vi "GigE Vision Set Packet Size.vi"(8 "error in (no error)":errorcluster, 10 "Packet Size":i32, 11 "Camera in":refnum<class "Camera.lvclass">) -> (0 "error out":errorcluster, 3 "Camera":refnum<class "Camera.lvclass">)   [LabVIEW 2020, in "Camera.lvclass"]
doc: "Specifies the stream packet size, in bytes, to send on the selected channel for a GVSP transmitter or specifies the maximum packet size supported by a GVSP receiver.\n\nThis does not include data leader and data trailer and the last data packet which might be of smaller size (since packet size is not necessarily a multiple of block size for stream channel). Negative packet_size is ignored."
uses:
  Camera.lvclass
  Camera.lvclass/Camera.ctl
  bin/gindustrialcam_32-1.dll
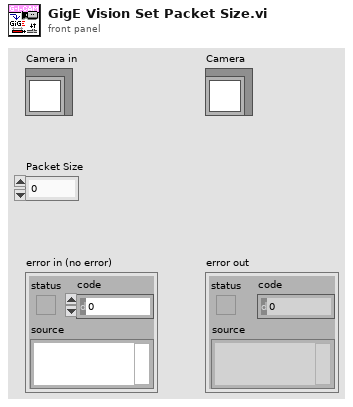
[diagram p1: front panel]
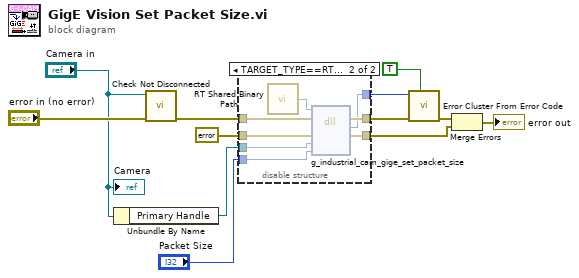
[diagram p0: block diagram]
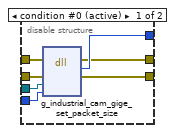
[diagram p2: hidden frame]
diagram:
  n1 = Unbundle By Name("Camera in") -> ("Primary Handle"=w2:refnum<data-value>)
  n2 = call "Check Not Disconnected.vi"("error in (no error)"="error in (no error)", "Camera in"="Camera in") -> ("error out"=w10:errorcluster)  [unwired: 9 in]
  n3 = disable-structure shown="TARGET_TYPE==RT&&OS==Linux" {
    disable-tunnel: w10 -> [w19 w26]
    disable-tunnel: errorcluster {"status"=FALSE, "code"=0, "source"=""} ("error constant") -> [w18 w25]
    disable-tunnel: [w17 w20] -> w7
    disable-tunnel: [w16 w21] -> w5
    disable-tunnel: [w15 w22] -> w4
    disable-tunnel: w2 -> [w14 w24]
    disable-tunnel: "Packet Size" -> [w13 w23]
    frame condition #0 (active) {
      n4 = dll-call lib="C:/serenial/lib/g-industrial-camera/LabVIEW/g_industrial_cam/bin/gindustrialcam_*-1.*" fn="g_industrial_cam_gige_set_packet_size"(error in=w19, "err"=w18, "edvr"=w14, "size"=w13) -> (error out=w15:errorcluster, "Mg_Error"=w16:i32, "err"=w17:errorcluster)  [unwired: 4 in, 1 out]
    }
    frame condition #1 {
      n5 = call "RT Shared Binary Path.vi"() -> ("Path"=w27:path)
      n6 = dll-call lib="?" fn="g_industrial_cam_gige_set_packet_size"(path in=w27, error in=w26, "err"=w25, "edvr"=w24, "size"=w23) -> (error out=w22:errorcluster, "Mg_Error"=w21:i32, "err"=w20:errorcluster)  [unwired: 3 in, 1 out]
    }
  }
  n7 = call <vilib>:"Error Cluster From Error Code.vi"("show call chain? (False)"=TRUE, "error in (no error)"=w4, "error code (0)"=w5) -> ("error out"=w6:errorcluster)  [unwired: 6 in]
  n8 = Merge Errors(w6, w7) -> (→"error out":errorcluster)
  "Camera" <- "Camera in"
